vi "Estimate b.vi"(8 "Beta":dbl[][](array[numeric]), 9 "Alpha":dbl[][](array[numeric]), 10 "Observed states":i32[](array[numeric]), 11 "HMM Cluster":T1) -> (3 "Estimated b":dbl[][](array[numeric]))   [LabVIEW 2014, in "HMM.lvlib"]
doc: "Estimates the confusion matrix (b) with the input HMM model."
uses:
  HMM.lvlib
  Control/HMM Cluster.ctl
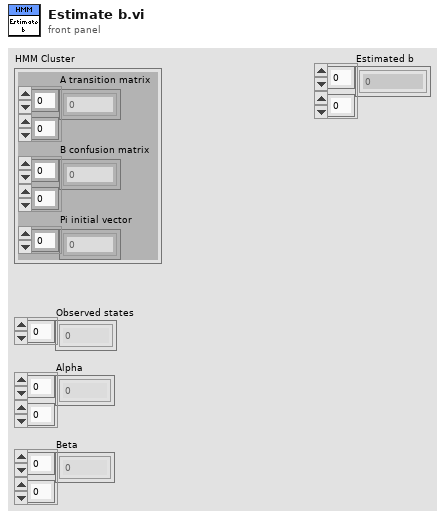
[diagram p1: front panel]
types:
  T1 = typedef "HMM.lvlib/HMM Cluster.ctl" = cluster{"A transition matrix":dbl[][], "B confusion matrix":dbl[][], "Pi initial vector":dbl[]}
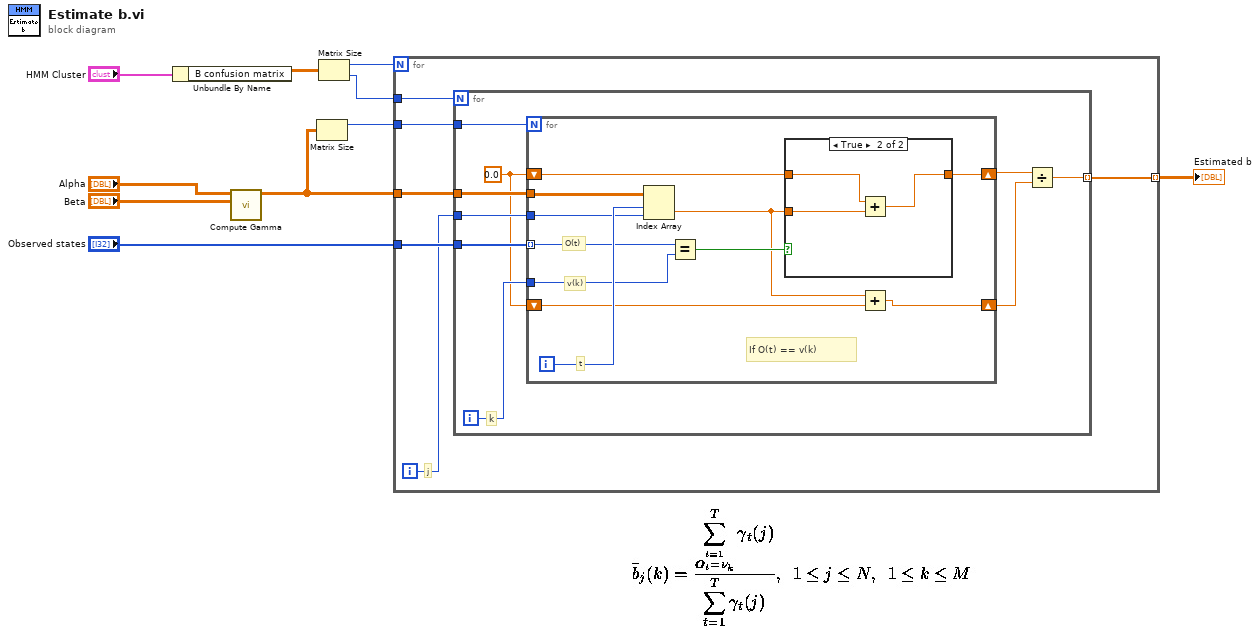
[diagram p0: block diagram]
diagram:
  n1 = Unbundle By Name("HMM Cluster") -> ("B confusion matrix"=w10:dbl[][])
  n2 = call "Compute Gamma.vi"("Beta"="Beta", "Alpha"="Alpha") -> ("Gamma"=w7:dbl[][])  [unwired: 9 in]
  n3 = Matrix Size(0:w7) -> (1:w6:i32)  [unwired: 1 out]
  n4 = Matrix Size(0:w10) -> (1:w9:i32, 2:w8:i32)
  n5 = for {
    N: w9 -> [_]
    tunnel: w7 -> [w16]
    tunnel: "Observed states" -> [w15]
    tunnel: [w13] -> w3 mode=indexing
    tunnel: w8 -> [w12]
    tunnel: w6 -> [w11]
    i -> [w14]
    # "j"
    n6 = for {
      N: w12 -> [_]
      tunnel: w16 -> [w25]
      tunnel: w15 -> [w24]
      tunnel: w14 -> [w22]
      tunnel: [w18] -> w13 mode=indexing
      tunnel: w11 -> [w17]
      i -> [w23]
      w21 = 0.0
      # "k"
      n7 = for {
        N: w17 -> [_]
        tunnel: w25 -> [w36]
        tunnel: w24 -> [w33] mode=indexing
        tunnel: w23 -> [w32]
        tunnel: w22 -> [w34]
        shift-right: [w30] -> w20
        shift-left: w21 -> [w29]
        shift-right: [w27] -> w19
        shift-left: w21 -> [w28]
        i -> [w35]
        # "If O(t) == v(k)"
        # "O(t)"
        # "v(k)"
        # "t"
        n8 = Index Array(array=w36, index (row)=w35, index (col)=w34) -> (element=w26:dbl)
        n9 = Equal?(x=w33, y=w32) -> (x = y?=w31:bool)
        n10 = case shown="True" w31 {
          tunnel: w26 -> [_ w40]
          tunnel: [w37 w38] -> w30
          tunnel: w29 -> [w37 w39]
          frame False {
          }
          frame True {
            n11 = Add(x=w39, y=w40) -> (x+y=w38:dbl)
          }
        }
        n12 = Add(x=w26, y=w28) -> (x+y=w27:dbl)
      }
      n13 = Divide(x=w20, y=w19) -> (x/y=w18:dbl)
    }
  }
  "Estimated b" <- w3
